vi "ProcessStopped_GET.vi"(8 "error in":errorcluster, 11 "server in":refnum<class "RT FlexRIO Server TCP.lvclass">) -> (0 "error out":errorcluster, 2 "state request":refnum<user-event>, 3 "server out":refnum<class "RT FlexRIO Server TCP.lvclass">)   [LabVIEW 2017, in "RT FlexRIO Server TCP.lvclass"]
uses:
  RT FlexRIO Server TCP.lvclass
  Public/State.ctl
  RT FlexRIO Server TCP.lvclass/RT FlexRIO Server TCP.ctl
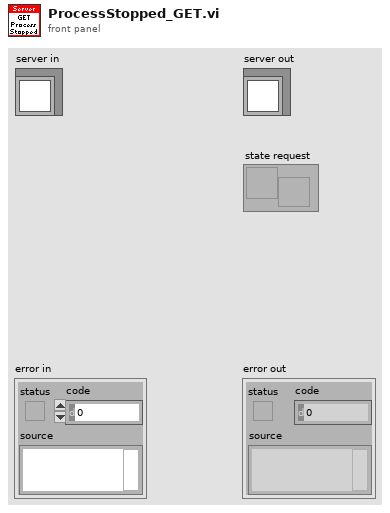
[diagram p1: front panel]
types:
  T1 = typedef "RT FlexRIO Server TCP.lvclass/SessionData.ctl" = cluster{"listener":refnum<k5>, "connection":refnum<k5>, "state":T2, "incoming":refnum<queue>, "outgoing":refnum<queue>, "state request":refnum<user-event>, "state changed":refnum<user-event>}
  T2 = typedef "RT FlexRIO Server TCP.lvclass/connection state.ctl" = enum16{"started", "connected", "stopped"}
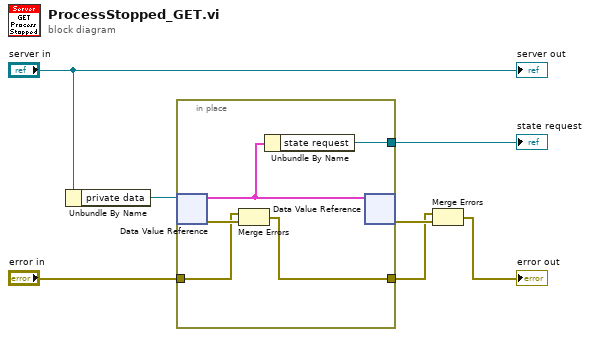
[diagram p0: block diagram]
diagram:
  n1 = Unbundle By Name("server in") -> ("private data"=w7:refnum<data-value>)
  n2 = in-place {
    in-place-border: "error in" -> [w8]
    in-place-border: [w12] -> w4
    in-place-border: [w10] -> w1
    n3 = in-place-dvr #1(w7) -> (w11:T1, w9:errorcluster)
    n4 = Merge Errors(w8, w9) -> (w12:errorcluster)
    n5 = Unbundle By Name(w11) -> ("state request"=w10:refnum<user-event>)
    n6 = in-place-dvr #1(w11) -> (w5:errorcluster)  [unwired: 1 out]
  }
  "state request" <- w1
  n7 = Merge Errors(w4, w5) -> (→"error out":errorcluster)
  "server out" <- "server in"
